vi "Close Sessions.vi"(8 "error in (no error)":errorcluster, 11 "Panel State Data In":T1={"FGEN Resource"="", "DAQmx Tasks Session"={"DO Task"="", "Ctr0 Task"=""}, "Scope Resource"="", "FGEN Enabled?"=FALSE, "DAQ Enabled?"=FALSE, "Scope Enabled?"=FALSE, "Max Total FGEN Wfm Duration (s)"=0.0, "FGEN-DAQ Routing"={"FGEN Start Trigger"="", "DAQ Trig Line"=""}, "Scope Recording Settings"={"Number of Records"=0, "Channels Per Record"=1, "Plot Names"=[], "Fetch Timeout"=0.0, "Channel List"=""}} {"Scope Recording Settings"."Fetch Timeout" format="%.2f"}) -> (0 "error out":errorcluster, 3 "Panel State Data Out":T1={"FGEN Resource"="", "DAQmx Tasks Session"={"DO Task"="", "Ctr0 Task"=""}, "Scope Resource"="", "FGEN Enabled?"=FALSE, "DAQ Enabled?"=FALSE, "Scope Enabled?"=FALSE, "Max Total FGEN Wfm Duration (s)"=0.0, "FGEN-DAQ Routing"={"FGEN Start Trigger"="", "DAQ Trig Line"=""}, "Scope Recording Settings"={"Number of Records"=0, "Channels Per Record"=1, "Plot Names"=[], "Fetch Timeout"=0.0, "Channel List"=""}} {"Scope Recording Settings"."Fetch Timeout" format="%.2f"})   [LabVIEW 2025]
uses:
  Typedef/Test Panel State Data.ctl
  Typedef/Scope Recording Settings.ctl
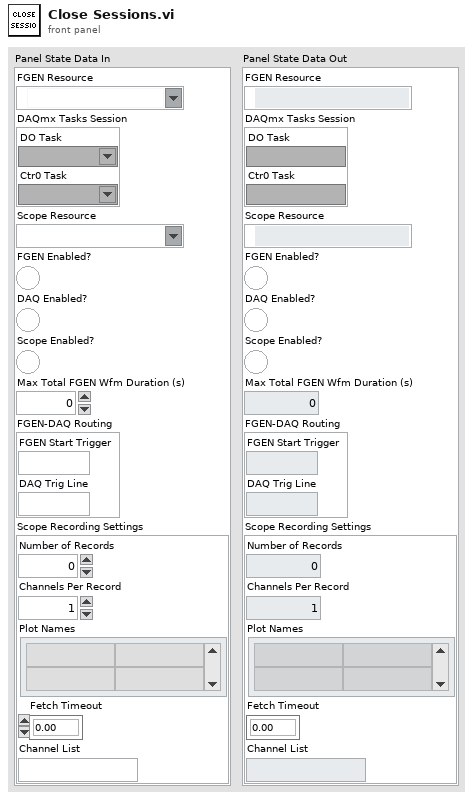
[diagram p1: front panel]
types:
  T1 = typedef "Test Panel State Data.ctl" = cluster{"FGEN Resource":refnum<k15>, "DAQmx Tasks Session":cluster{"DO Task":refnum<k21>, "Ctr0 Task":refnum<k21>}, "Scope Resource":refnum<k15>, "FGEN Enabled?":bool, "DAQ Enabled?":bool, "Scope Enabled?":bool, "Max Total FGEN Wfm Duration (s)":dbl, "FGEN-DAQ Routing":cluster{"FGEN Start Trigger":string, "DAQ Trig Line":string}, "Scope Recording Settings":T2}
  T2 = typedef "Scope Recording Settings.ctl" = cluster{"Number of Records":i32, "Channels Per Record":i32, "Plot Names":string[][], "Fetch Timeout":dbl, "Channel List":string}
  T3 = cluster{"DO Task":refnum<k21>, "Ctr0 Task":refnum<k21>}
  T4 = cluster{"FGEN Start Trigger":string, "DAQ Trig Line":string}
  T5 = enum16{"Reset", "Start", "Read", "Pause", "Resume"}
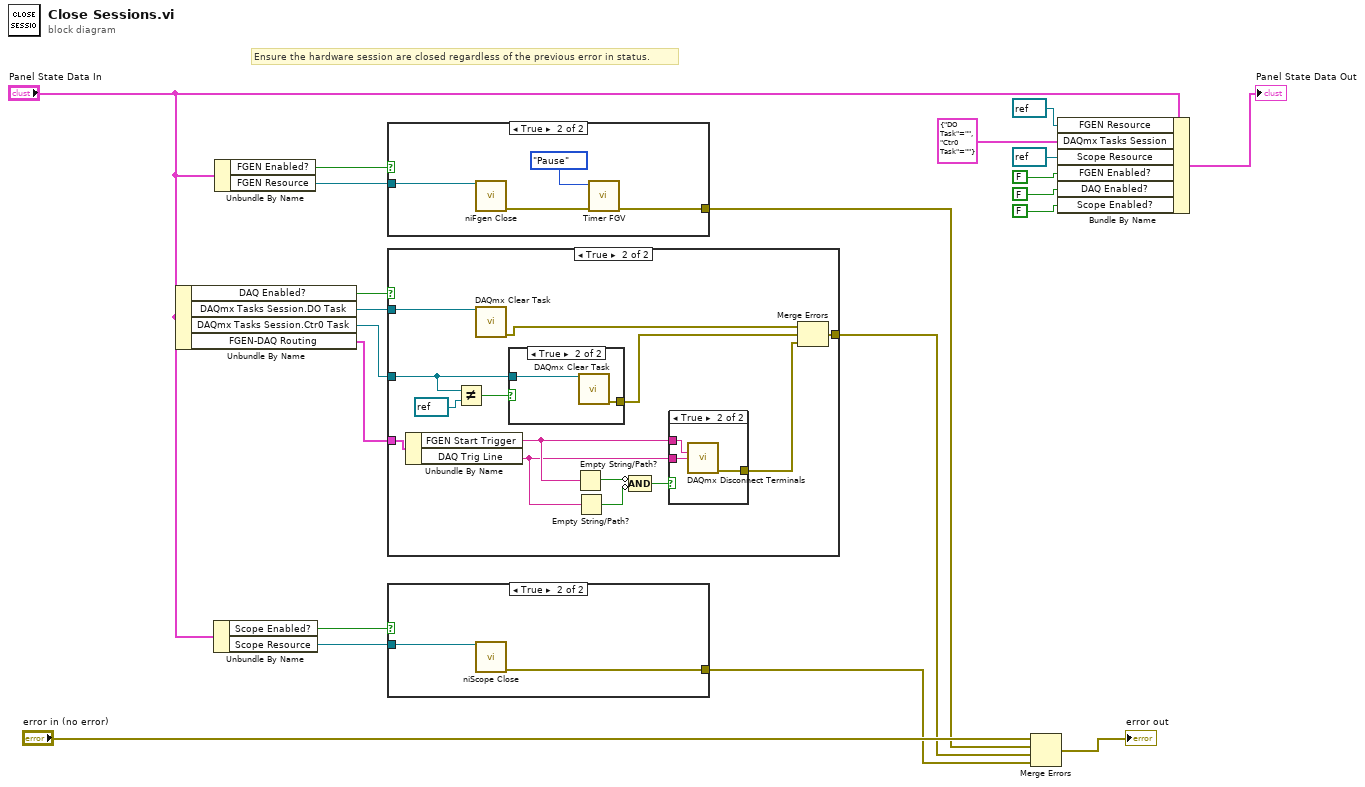
[diagram p0: block diagram]
diagram:
  # "Ensure the hardware session are closed regardless of the previous error in status."
  n1 = Unbundle By Name("Panel State Data In") -> ("DAQ Enabled?"=w17:bool, "DAQmx Tasks Session.DO Task"=w18:refnum<k21>, "DAQmx Tasks Session.Ctr0 Task"=w3:refnum<k21>, "FGEN-DAQ Routing"=w1:T4)
  n2 = Unbundle By Name("Panel State Data In") -> ("Scope Enabled?"=w16:bool, "Scope Resource"=w15:refnum<k15>)
  n3 = Unbundle By Name("Panel State Data In") -> ("FGEN Enabled?"=w20:bool, "FGEN Resource"=w19:refnum<k15>)
  n4 = case shown="True" w20 {
    tunnel: w19 -> [_ w25]
    tunnel: [_ w23] -> w12
    frame False {
    }
    frame True {
      n5 = call <instrlib>:"niFgen Close.vi"("Instrument Handle"=w25) -> ("error out"=w24:errorcluster)  [unwired: 10 in]
      n6 = call "Timer FGV.vi"("error in (no error)"=w24, "Timer mode"=T5."Pause") -> ("error out"=w23:errorcluster)  [unwired: 6 in, 3 out]
    }
  }
  n7 = case shown="True" w17 {
    tunnel: w18 -> [_ w39]
    tunnel: [_ w32] -> w11
    tunnel: w3 -> [_ w28]
    tunnel: w1 -> [_ w37]
    frame False {
    }
    frame True {
      n8 = Unbundle By Name(w37) -> ("FGEN Start Trigger"=w34:string, "DAQ Trig Line"=w33:string)
      n9 = Not Equal?(x=w28, y=refnum<k21> refnum) -> (x != y?=w26:bool)
      n10 = call <vilib>:"DAQmx Clear Task.vi"("task in"=w39) -> ("error out"=w31:errorcluster)  [unwired: 14 in]
      n11 = case shown="True" w26 {
        tunnel: [_ w41] -> w38
        tunnel: w28 -> [_ w40]
        frame False {
        }
        frame True {
          n12 = call <vilib>:"DAQmx Clear Task.vi"("task in"=w40) -> ("error out"=w41:errorcluster)  [unwired: 14 in]
        }
      }
      n13 = Empty String/Path?(string/path=w34) -> (empty?=w36:bool)
      n14 = Empty String/Path?(string/path=w33) -> (empty?=w35:bool)
      n15 = Compound Arithmetic op=AND(invert w36, invert w35) -> (w29:bool)
      n16 = case shown="True" w29 {
        tunnel: w34 -> [_ w44]
        tunnel: w33 -> [_ w43]
        tunnel: [_ w42] -> w30
        frame False {
        }
        frame True {
          n17 = call <vilib>:"DAQmx Disconnect Terminals.vi"("source terminal"=w44, "destination terminal"=w43) -> ("error out"=w42:errorcluster)  [unwired: 13 in]
        }
      }
      n18 = Merge Errors(w31, w38, w30) -> (w32:errorcluster)
    }
  }
  n19 = case shown="True" w16 {
    tunnel: w15 -> [_ w45]
    tunnel: [_ w46] -> w10
    frame False {
    }
    frame True {
      n20 = call <instrlib>:"niScope Close.vi"("instrument handle"=w45) -> ("error out"=w46:errorcluster)  [unwired: 14 in]
    }
  }
  n21 = Merge Errors("error in (no error)", w12, w11, w10) -> (→"error out":errorcluster)
  n22 = Bundle By Name(cluster="Panel State Data In", "FGEN Resource"=refnum<k15> refnum, "DAQmx Tasks Session"=T3 {"DO Task"="", "Ctr0 Task"=""}, "Scope Resource"=refnum<k15> refnum, "FGEN Enabled?"=FALSE, "DAQ Enabled?"=FALSE, "Scope Enabled?"=FALSE) -> (→"Panel State Data Out":T1)
